vi "StreamEngine.Main.Stream.BusStatus.Process.vi"(8 "error in (no error)":errorcluster, 10 "Stream Connection":bool, 11 "State":T1 {"fault code" format="%08x"; "last error" items=["None", "Stuff", "Form", "Ack", "Bit1", "Bit0", "CRC"]; "communication state" items=["Error Active", "Error Passive", "Bus Off", "Init"]}) -> (0 "error out":errorcluster, 2 "Warning":bool, 3 "State":string)   [LabVIEW 2025, in "XNET Bus Monitor Client.lvlib"]
uses:
  XNET Bus Monitor Client.lvlib
  <vilib>/xnet/xnet.llb/XNET CAN Comm.ctl
  <vilib>/xnet/xnet.llb/XNET CAN Comm State.ctl
  <vilib>/xnet/xnet.llb/XNET CAN Last Err.ctl
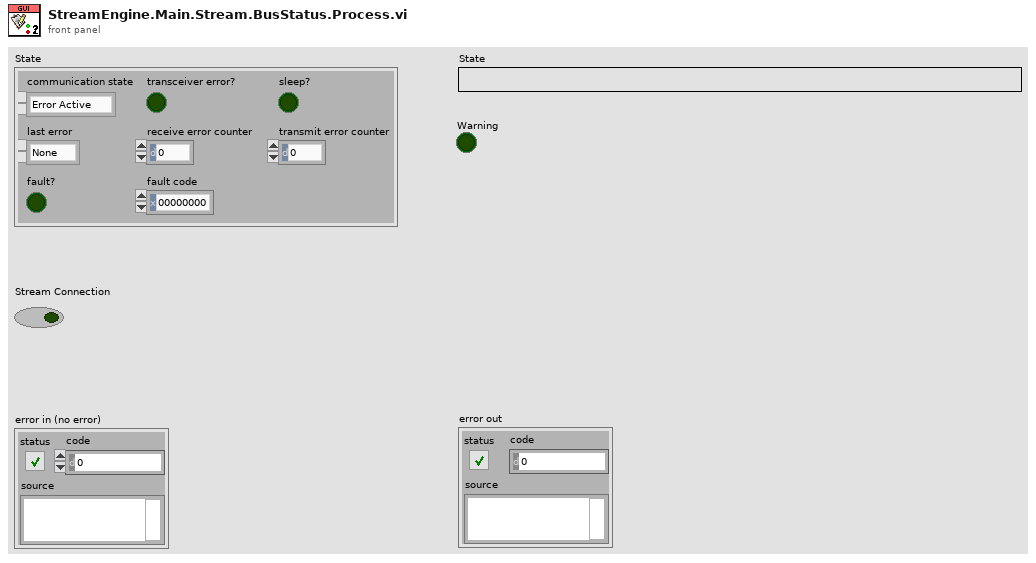
[diagram p1: front panel]
types:
  T1 = typedef "XNET CAN Comm.ctl" = cluster{"fault code":i32, "fault?":bool, "communication state":T2, "last error":T3, "receive error counter":u8, "transmit error counter":u8, "transceiver error?":bool, "sleep?":bool}
  T2 = typedef "XNET CAN Comm State.ctl" = u8
  T3 = typedef "XNET CAN Last Err.ctl" = u8
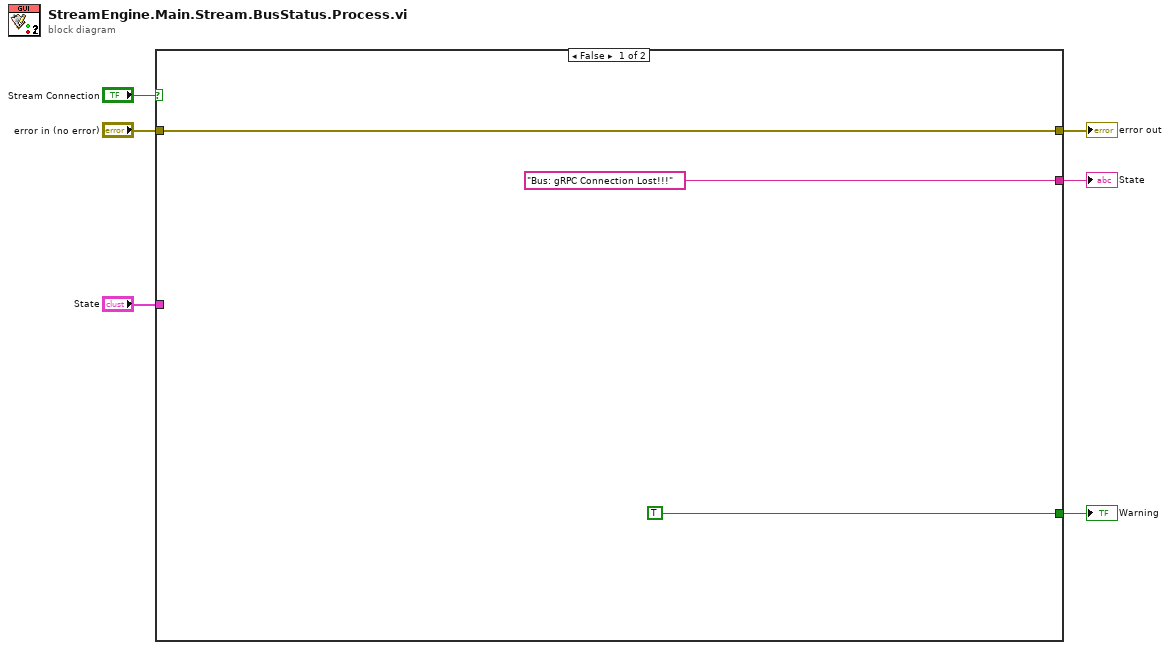
[diagram p0: block diagram]
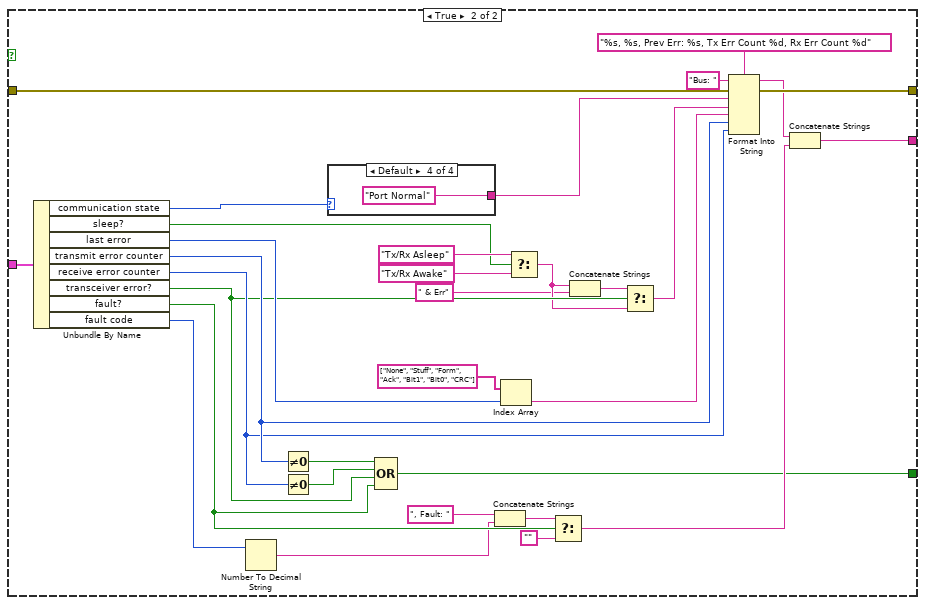
[diagram p2: hidden frame]
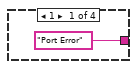
[diagram p3: hidden frame]
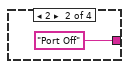
[diagram p4: hidden frame]
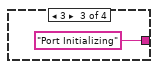
[diagram p5: hidden frame]
diagram:
  n1 = case shown="False" "Stream Connection" {
    tunnel: [w8 w41] -> w6
    tunnel: "error in (no error)" -> [w8 w40]
    tunnel: "State" -> [_ w33]
    tunnel: ["Bus: gRPC Connection Lost!!!" w16] -> w3
    tunnel: [TRUE w10] -> w1
    frame False {
    }
    frame True {
      n2 = Unbundle By Name(w33) -> ("communication state"=w34:T2, "sleep?"=w35:bool, "last error"=w31:T3, "transmit error counter"=w29:u8, "receive error counter"=w28:u8, "transceiver error?"=w24:bool, "fault?"=w23:bool, "fault code"=w22:i32)
      n3 = Number To Decimal String(number=w22) -> (decimal integer string=w20:string)  [unwired: 1 in]
      n4 = Not Equal To 0?(x=w29) -> (x != 0?=w26:bool)
      n5 = Not Equal To 0?(x=w28) -> (x != 0?=w27:bool)
      n6 = case shown="Default" w34 {
        tunnel: ["Port Error" "Port Off" "Port Initializing" "Port Normal"] -> w39
        frame 1 {
        }
        frame 2 {
        }
        frame 3 {
        }
        frame Default {
        }
      }
      n7 = Compound Arithmetic op=OR(w26, w27, w24, w23) -> (w10:bool)
      n8 = Concatenate Strings(", Fault: " ("t"), w20) -> (w19:string)
      n9 = Index Array(array=string[] ["None", "Stuff", "Form", "Ack", "Bit1", "Bit0", "CRC"] ("Strings []"), index=w31) -> (element=w30:string)
      n10 = Select(t="Tx/Rx Asleep", s=w35, f="Tx/Rx Awake") -> (s? t:f=w14:string)
      n11 = Select(t=w19, s=w23, f="") -> (s? t:f=w15:string)
      n12 = Concatenate Strings(w14, " & Err" ("t")) -> (w12:string)
      n13 = Select(t=w12, s=w24, f=w14) -> (s? t:f=w25:string)
      n14 = Format Into String(format string="%s, %s, Prev Err: %s, Tx Err Count %d, Rx Err Count %d", initial string="Bus: ", error in=w40, w39, w25, w30, w29, w28) -> (resulting string=w17:string, error out=w41:errorcluster)
      n15 = Concatenate Strings(w17, w15) -> (w16:string)
    }
  }
  "error out" <- w6
  "State" <- w3
  "Warning" <- w1
